vi "FT.vi"(3 "Retardo":dbl min=0.0 format="%#_3g", 4 "Denominador":dbl[](array[numeric]), 5 "Numerador":dbl[](array[numeric])) -> (0 "C":dbl[](array[numeric]), 1 "B":dbl[](array[numeric]), 2 "A":T1)   [LabVIEW 2019]
uses:
  <vilib>/Analysis/Matrix/Datatypes/RealMatrix.ctl
  <vilib>/Analysis/7linalg.llb/Create Special Real Matrix.vi
  <vilib>/Analysis/NI_AALPro.lvlib
  <vilib>/Analysis/Matrix/NI_Matrix.lvlib
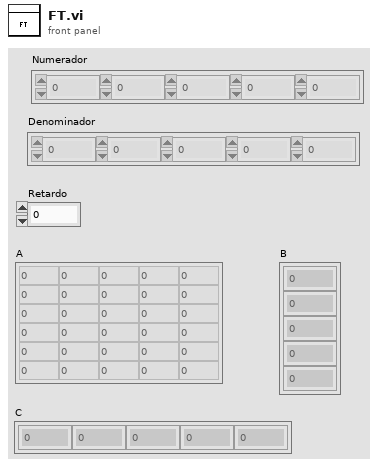
[diagram p1: front panel]
types:
  T1 = typedef "NI_Matrix.lvlib/RealMatrix.ctl" = dbl[][]
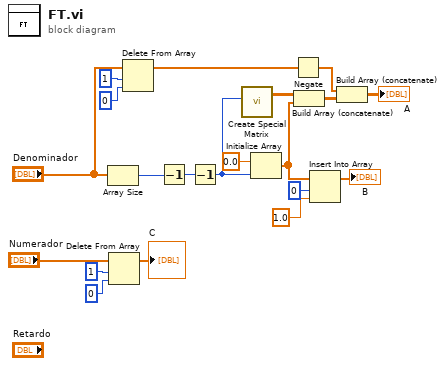
[diagram p0: block diagram]
diagram:
  n1 = Array Size(array="Denominador") -> (size(s)=w20:i32)
  n2 = Delete From Array(array="Numerador", length=1 ("index"), index=0 ("length")) -> (array with subset deleted=→"C":dbl[])  [unwired: 1 out]
  n3 = Delete From Array(array="Denominador", length=1 ("index"), index=0 ("length")) -> (array with subset deleted=w11:dbl[])  [unwired: 1 out]
  n4 = Decrement(x=w20) -> (x-1=w9:i32)
  n5 = Decrement(x=w9) -> (x-1=w19:i32)
  n6 = call-poly <vilib>:"Create Special Matrix.vi"("matrix size"=w19) -> ("Special Matrix"=w17:T1)  [unwired: 4 in, 1 out]
  n7 = Initialize Array(0.0 ("element"), w19) -> (w8:dbl[])
  n8 = Negate(x=w11) -> (-x=w10:dbl[])
  n9 = Build Array (concatenate)(w17, w8) -> (w13:T1)
  n10 = Insert Into Array(array=w8, index=0, new element=1.0 ("new element/subarray")) -> (→"B":dbl[])
  n11 = Build Array (concatenate)(w10, w13) -> (→"A":T1)
